vi "rtin_controlRealTimeInMode.vi"(7 "Set":bool, 8 "error in":errorcluster, 9 "mode":i32, 10 "axis in":u8, 11 "connection ID":refnum<k5>) -> (0 "error out":errorcluster, 1 "mode out":i32, 2 "axis out":i32, 3 "connection ID":refnum<k5>)   [LabVIEW 2016, in "AMC_VIs.lvlib"]
doc: "This function sets or retrieves the real time input mode for the selected axis."
uses:
  AMC_VIs.lvlib
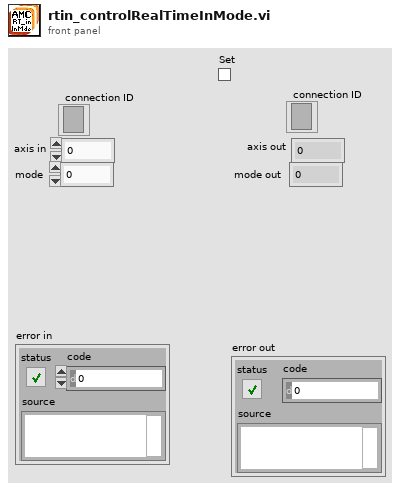
[diagram p1: front panel]
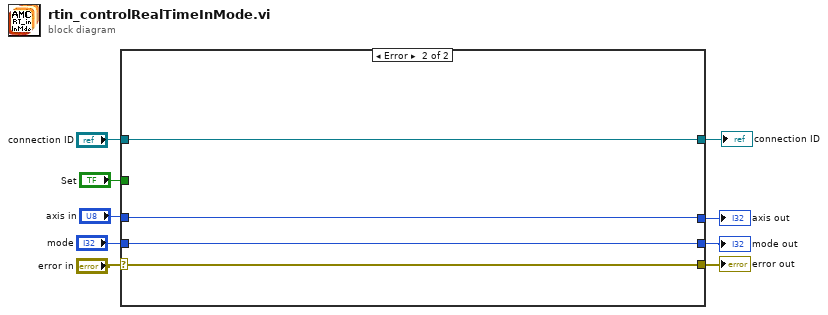
[diagram p0: block diagram]
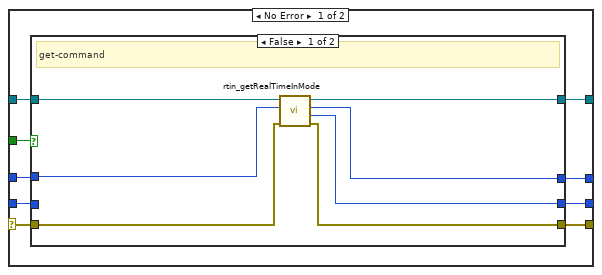
[diagram p2: hidden frame]
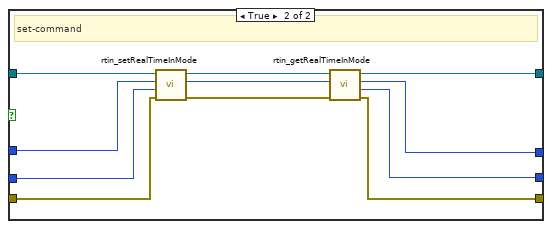
[diagram p3: hidden frame]
diagram:
  n1 = case shown="Error" "error in" {
    selector: "error in" -> [w14 w40]
    tunnel: "axis in" -> [w18 w38]
    tunnel: [w12 w40] -> w8
    tunnel: "mode" -> [w16 w39]
    tunnel: [w13 w39] -> w3
    tunnel: "Set" -> [w15 _]
    tunnel: [w11 w37] -> w6
    tunnel: "connection ID" -> [w17 w37]
    tunnel: [w10 w38] -> w1
    frame No Error {
      n2 = case shown="False" w15 {
        tunnel: w17 -> [w25 w32]
        tunnel: w18 -> [w19 w27]
        tunnel: w16 -> [_ w26]
        tunnel: w14 -> [w24 w33]
        tunnel: [w20 w29] -> w13
        tunnel: [w23 w31] -> w12
        tunnel: [w22 w30] -> w11
        tunnel: [w21 w28] -> w10
        frame False {
          # "get-command"
          n3 = call "rtin_getRealTimeInMode.vi"("error in"=w24, "axis"=w19, "connection ID"=w25) -> ("error out"=w23:errorcluster, "mode"=w20:i32, "axis_out"=w21:i32, "connection ID"=w22:refnum<k5>)  [unwired: 5 in]
        }
        frame True {
          # "set-command"
          n4 = call "rtin_setRealTimeInMode.vi"("error in"=w33, "mode"=w26, "axis"=w27, "connection ID"=w32) -> ("error out"=w34:errorcluster, "axis_out"=w36:i32, "connection ID"=w35:refnum<k5>)  [unwired: 5 in]
          n5 = call "rtin_getRealTimeInMode.vi"("error in"=w34, "axis"=w36, "connection ID"=w35) -> ("error out"=w31:errorcluster, "mode"=w29:i32, "axis_out"=w28:i32, "connection ID"=w30:refnum<k5>)  [unwired: 5 in]
        }
      }
    }
    frame Error {
    }
  }
  "error out" <- w8
  "axis out" <- w1
  "mode out" <- w3
  "connection ID" <- w6
